vi "VI Server_Set Tab Ctr Page by Page Label_Signaling.vi"(7 "TabCtr.Label":string="TESTs", 8 "error in":errorcluster, 9 "Page.Label":string, 11 "VI Server Cluster":T1={"VI Ref"=refnum, "Refs"=[], "Labels"=["Label", "Size", "Font", "Heght", "Width", "Ledding Denominator", "Ledding Nominator", "Label Number", "Microstep Resolution", "X", "Y", "Z", "Italic?", "Underlined?"]}) -> (0 "error out":errorcluster, 3 "VI Server Cluster.DUP":T1={"VI Ref"=refnum, "Refs"=[], "Labels"=["Label", "Size", "Font", "Heght", "Width", "Ledding Denominator", "Ledding Nominator", "Label Number", "Microstep Resolution", "X", "Y", "Z", "Italic?", "Underlined?"]})   [LabVIEW 2020, in "VI Server Toolkit LV2013.lvlib"]
doc: "Flips Tab Control page by its signaling value by the selected page name."
uses:
  VI Server Toolkit LV2013.lvlib
  VI Server Cluster.ctl
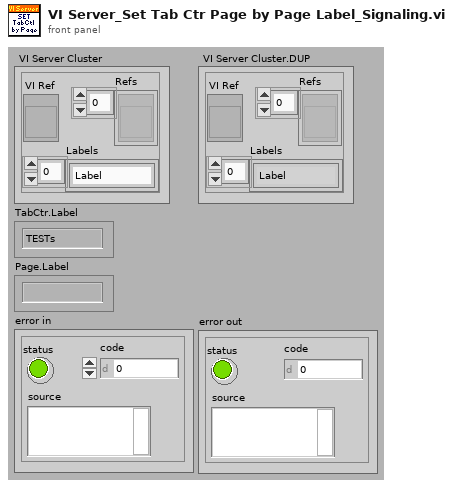
[diagram p1: front panel]
types:
  T1 = typedef "VI Server Toolkit LV2013.lvlib/VI Server Cluster.ctl" = cluster{"VI Ref":refnum<vi>, "Refs":refnum<vi>[], "Labels":string[]}
  T2 = enum32{"Input Signal", "Output Signal", "Phase Error", "T-Skew", "Cycle-To-Cycle Jitter", "Non-Repetitive Jitter", "Signal Spectrum"}
  T3 = typedef "VI Server_RefsCluster.ctl" = cluster{"Labels":string[], "Refs":refnum<vi>[], "VI Ref":refnum<vi>}
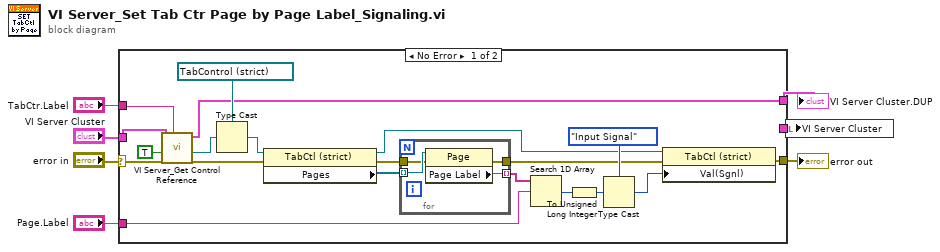
[diagram p0: block diagram]
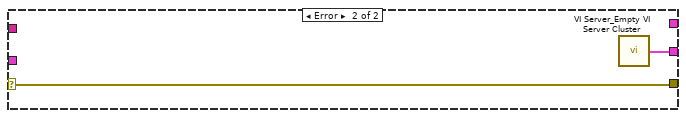
[diagram p2: hidden frame]
diagram:
  n1 = case shown="No Error" "error in" {
    selector: "error in" -> [w12 w33]
    tunnel: [w27 w33] -> w7
    tunnel: "Page.Label" -> [w20 _]
    tunnel: "TabCtr.Label" -> [w9 _]
    tunnel: "VI Server Cluster" -> [w13 _]
    tunnel: [w11 _] -> w2
    tunnel: [_ w32] -> w1
    frame No Error {
      n2 = call "VI Server_Get Control Reference.vi"("Label"=w9, "error in"=w12, "Single Instance (T)"=TRUE, "VI Server Cluster"=w13) -> ("error out"=w16:errorcluster, "Control Reference (Generic)"=w10:refnum<vi>, "VI Server Cluster.DUP"=w11:T3)  [unwired: 4 in, 1 out]
      n3 = Type Cast(type=refnum<vi> refnum ("Tabref"), x=w10) -> (*(type *) &x=w15:refnum<vi>)
      n4 = property class="TabCtl (strict)"(reference=w15, error in=w16) -> (reference out=w22:refnum<vi>, error out=w18:errorcluster, "Pages"=w17:refnum<vi>[])
      n5 = for {
        tunnel: w17 -> [w31] mode=indexing
        tunnel: w18 -> [w30]
        tunnel: [w29] -> w21
        tunnel: [w28] -> w19 mode=indexing
        n6 = property class="Page"(reference=w31, error in=w30) -> (error out=w29:errorcluster, "Page Label"=w28:string)  [unwired: 1 out]
      }
      n7 = Search 1D Array(1D array=w19, element=w20) -> (index of element=w23:i32)  [unwired: 1 out]
      n8 = To Unsigned Long Integer(number=w23) -> (unsigned 32bit integer=w24:u32)
      n9 = Type Cast(type=T2."Input Signal" ("Value"), x=w24) -> (*(type *) &x=w26:T2)
      n10 = property class="TabCtl (strict)"(reference=w22, error in=w21, "Val(Sgnl)"=w26) -> (error out=w27:errorcluster)  [unwired: 1 out]
    }
    frame Error {
      n11 = call "VI Server_Empty VI Server Cluster.vi"() -> ("VI Server Cluster"=w32:T3)  [unwired: 7 in]
    }
  }
  "error out" <- w7
  "VI Server Cluster.DUP" <- w2
  n12 = local write "VI Server Cluster"(w1) -> ()
